vi "Initialize.vi"(7 "Limit Name":string="Setpoint.ch%d.SP", 8 "error in":errorcluster, 9 "Number of Channels":u32=1, 10 "Instance Name":string="PluginName", 11 "Limit in":refnum<class "Limit.lvclass">) -> (0 "error out":errorcluster caption="error in", 3 "Limit out":refnum<class "Limit.lvclass">)   [LabVIEW 2023, in "Limit.lvclass"]
uses:
  Limit.lvclass
  Limit.lvclass/Limit.ctl
  <vilib>/ADAS Replay HIL/Channels/Tag Wrapper/Polymorphic/Open Consumer Tag (Double).vi
  <vilib>/ADAS Replay HIL/Channels/Tag Wrapper/Polymorphic/Set Default Value (Double).vi
  <vilib>/ADAS Replay HIL/Channels/Tag Wrapper/Polymorphic/Open Consumer Tag (Double).vi/bacb721e-673a-491a-accd-959f2e1f334e.vi
  <vilib>/ADAS Replay HIL/Channels/Tag Wrapper/Polymorphic/Set Default Value (Double).vi/228e99de-6fcf-414d-86fc-dc277c7b351f.vi
  <vilib>/ADAS Replay HIL/Channels/Tag Wrapper/Polymorphic/Open Consumer Tag (Double).vi/bacb721e-673a-491a-accd-959f2e1f334e.vi/c28b0ead-42ad-4072-80a2-aca7f2bd7ce3.vi
  <vilib>/ADAS Replay HIL/Channels/Tag Wrapper/Polymorphic/Set Default Value (Double).vi/228e99de-6fcf-414d-86fc-dc277c7b351f.vi/4bc1c15b-36ab-481f-b8dd-c64075ce723a.vi
  <vilib>/ADAS Replay HIL/AdasHilServices/AdasHilServices Fill In Error Info Ex.vi
  <vilib>/ADAS Replay HIL/Channels/Tag Wrapper/Tag Wrapper.lvlib
  Utilities/Utilities.lvlib
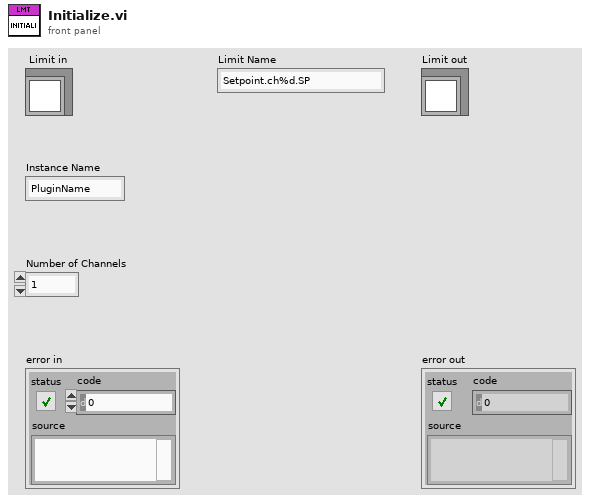
[diagram p1: front panel]
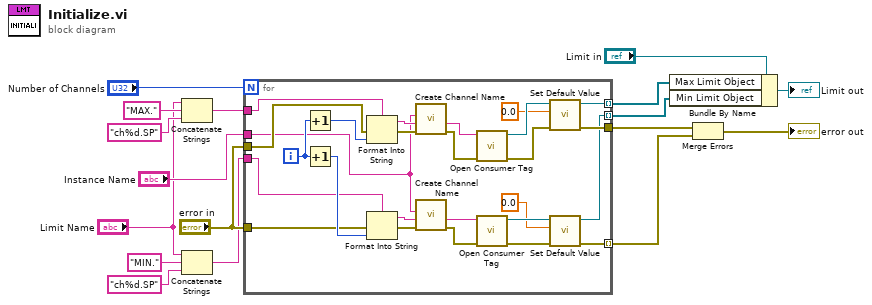
[diagram p0: block diagram]
diagram:
  n1 = Concatenate Strings("Limit Name", "MAX." ("string"), "ch%d.SP" ("string")) -> (w5:string)
  n2 = Concatenate Strings("Limit Name", "MIN." ("string"), "ch%d.SP" ("string")) -> (w1:string)
  n3 = for {
    N: "Number of Channels" -> [_]
    tunnel: [w37] -> w8
    tunnel: [w39] -> w15 mode=indexing
    tunnel: "error in" -> [w35]
    tunnel: "Instance Name" -> [w18]
    tunnel: w5 -> [w34]
    tunnel: "error in" -> [w27]
    tunnel: [w26] -> w10 mode=indexing
    tunnel: [w25] -> w9 mode=indexing
    tunnel: w1 -> [w19]
    i -> [w20]
    n4 = Increment(x=w20) -> (x+1=w43:i32)
    n5 = Increment(x=w20) -> (x+1=w33:i32)
    n6 = Format Into String(format string=w34, error in=w35, w43) -> (resulting string=w42:string, error out=w22:errorcluster)  [unwired: 1 in]
    n7 = Format Into String(format string=w19, error in=w27, w33) -> (resulting string=w32:string, error out=w21:errorcluster)  [unwired: 1 in]
    n8 = call "Create Channel Name.vi"("error in"=w22, "Channel Name"=w42, "Plugin Name"=w18) -> ("error out"=w24:errorcluster, "Data Channel Name"=w41:string)  [unwired: 7 in]
    n9 = call "Create Channel Name.vi"("error in"=w21, "Channel Name"=w32, "Plugin Name"=w18) -> ("error out"=w23:errorcluster, "Data Channel Name"=w31:string)  [unwired: 7 in]
    n10 = call-poly <vilib>:"Open Consumer Tag.vi"("error in"=w24, "Channel Name"=w41) -> ("error out"=w38:errorcluster, "ADAS HIL Channel"=w40:refnum<k21>)  [unwired: 8 in]
    n11 = call-poly <vilib>:"Open Consumer Tag.vi"("error in"=w23, "Channel Name"=w31) -> ("error out"=w29:errorcluster, "ADAS HIL Channel"=w30:refnum<k21>)  [unwired: 8 in]
    n12 = call-poly <vilib>:"Set Default Value.vi"("error in"=w38, "Default Value"=0.0, "ADAS HIL Channel in"=w40) -> ("error out"=w37:errorcluster, "ADAS HIL Channel out"=w39:refnum<k21>)  [unwired: 7 in]
    n13 = call-poly <vilib>:"Set Default Value.vi"("error in"=w29, "Default Value"=0.0, "ADAS HIL Channel in"=w30) -> ("error out"=w25:errorcluster, "ADAS HIL Channel out"=w26:refnum<k21>)  [unwired: 7 in]
  }
  n14 = Bundle By Name(cluster="Limit in", "Max Limit Object"=w15, "Min Limit Object"=w10) -> (→"Limit out":refnum<class "Limit.lvclass">)
  n15 = Merge Errors(w8, w9) -> (→"error out":errorcluster)
